vi "Gyro Steer.vi"(7 "PID gains":T1={"proportional gain (Kc)"=1.0, "integral time (Ti, min)"=0.01, "derivative time (Td, min)"=0.0} {"derivative time (Td, min)" format="%.3f"; "integral time (Ti, min)" format="%.3f"; "proportional gain (Kc)" format="%.3f"}, 8 "Gyro Tolerance":dbl, 9 "X Min Output":dbl, 10 "X Max Output":dbl, 11 "Target Heading":dbl) -> (0 "Finished?":bool, 3 "X out":dbl)   [LabVIEW 2016]
uses:
  Common Code/PID Gains.ctl
  <vilib>/addons/control/pid/pid.llb/PID (DBL).vi
  <vilib>/addons/control/pid/NI_PID_pid.lvlib
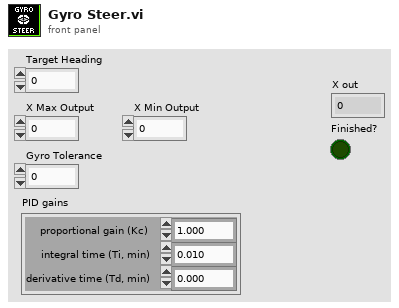
[diagram p1: front panel]
types:
  T1 = typedef "PID Gains.ctl" = cluster{"proportional gain (Kc)":dbl, "integral time (Ti, min)":dbl, "derivative time (Td, min)":dbl}
  T2 = cluster{"Yaw":dbl, "Roll":dbl, "Pitch":dbl, "Heading":dbl, "Fused Heading":dbl}
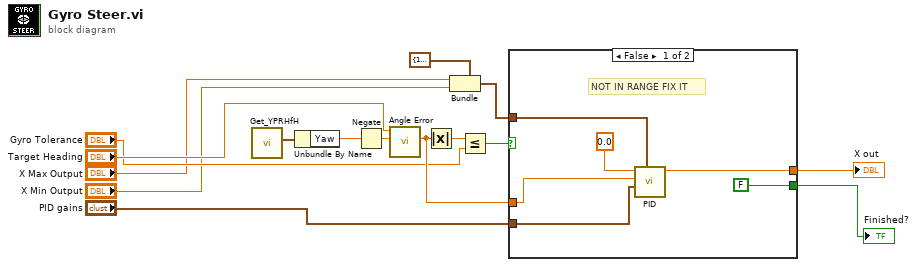
[diagram p0: block diagram]
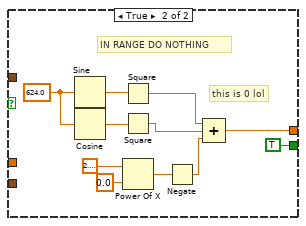
[diagram p2: hidden frame]
diagram:
  n1 = call <vilib>:"Get_YPRHfH.vi"() -> ("YRPHfH"=w15:T2)  [unwired: 11 in]
  n2 = Unbundle By Name(w15) -> ("Yaw"=w9:dbl)
  n3 = Negate(x=w9) -> (-x=w8:dbl)
  n4 = call "Angle Error.vi"("Angle"=w8, "Target Angle"="Target Heading") -> ("Error"=w12:dbl)  [unwired: 9 in]
  n5 = Absolute Value(x=w12) -> (abs(x)=w14:dbl)
  n6 = Bundle(cluster=cluster{"output high":dbl, "output low":dbl} {"output high"=100.0, "output low"=-100.0} ("output range"), "output high"="X Max Output", "output low"="X Min Output") -> (w10:cluster{"output high":dbl, "output low":dbl})
  n7 = Less Or Equal?(x=w14, y="Gyro Tolerance") -> (x <= y?=w13:bool)
  n8 = case shown="False" w13 {
    tunnel: w12 -> [w20 _]
    tunnel: w10 -> [w19 _]
    tunnel: "PID gains" -> [w18 _]
    tunnel: [w17 w23] -> w7
    tunnel: [FALSE TRUE] -> w2
    frame False {
      # "NOT IN RANGE FIX IT"
      n9 = call-poly <vilib>:"PID.vi"("output range"=w19, "PID gains"=w18, "process variable"=w20, "setpoint"=0.0) -> ("output"=w17:dbl)  [unwired: 6 in, 1 out]
    }
    frame True {
      w32 = 624.0 ("x")
      # "this is 0 lol"
      # "IN RANGE DO NOTHING"
      n10 = Sine(x=w32) -> (sin(x)=w31:dbl)
      n11 = Cosine(x=w32) -> (cos(x)=w30:dbl)
      n12 = Square(x=w31) -> (x^2=w29:dbl)
      n13 = Square(x=w30) -> (x^2=w28:dbl)
      n14 = Power Of X(1:0.0 ("x"), 2:2.718281828459045) -> (0:w25:dbl)
      n15 = Negate(x=w25) -> (-x=w24:dbl)
      n16 = Compound Arithmetic op=unknown(w29, w28, w24) -> (w23:dbl)
    }
  }
  "X out" <- w7
  "Finished?" <- w2
